vi "TrajectoryConfig_GetKinematicsMecanumDriveConstraint.vi"(11 "inTRAJECTORY_CONFIG":T1 {"End Velocity" format="%20.4f"; "StartVelocity" format="%20.4f"; "Max Acceleration" format="%20.4f"; "MaxVelocity" format="%20.4f"}) -> (1 "Constraint Exists":bool, 3 "Mecanum Drive Kinematics Constraint":T2={"Max Speed (M/S)"=0.0, "MECA_DRIVE_KINEMATICS"={"FrontLeft"={"X"=0.0, "Y"=0.0}, "FrontRight"={"X"=0.0, "Y"=0.0}, "RearLeft"={"X"=0.0, "Y"=0.0}, "RearRight"={"X"=0.0, "Y"=0.0}, "InverseKinematics"=[[0.0, 1.0, -1.0, 0.0], [0.0, 1.0, 1.0, 0.0], [0.0, 1.0, 1.0, 0.0], [0.0, 1.0, -1.0, 0.0]], "ForwardKinematics"=[[0.0, 1.0, -1.0, 0.0], [0.0, 1.0, 1.0, 0.0], [0.0, 1.0, 1.0, 0.0], [0.0, 1.0, -1.0, 0.0]], "PrevCoR"={"X"=0.0, "Y"=0.0}}} {"MECA_DRIVE_KINEMATICS"."PrevCoR"."Y" format="%14.3f"; "MECA_DRIVE_KINEMATICS"."PrevCoR"."X" format="%14.3f"; "MECA_DRIVE_KINEMATICS"."RearRight"."Y" format="%14.3f"; "MECA_DRIVE_KINEMATICS"."RearRight"."X" format="%14.3f"; "MECA_DRIVE_KINEMATICS"."RearLeft"."Y" format="%14.3f"; "MECA_DRIVE_KINEMATICS"."RearLeft"."X" format="%14.3f"; "MECA_DRIVE_KINEMATICS"."FrontRight"."Y" format="%14.3f"; "MECA_DRIVE_KINEMATICS"."FrontRight"."X" format="%14.3f"; "MECA_DRIVE_KINEMATICS"."FrontLeft"."Y" format="%14.3f"; "MECA_DRIVE_KINEMATICS"."FrontLeft"."X" format="%14.3f"; "Max Speed (M/S)" format="%20.4f"})   [LabVIEW 2019, in "Trajectory_Library.lvlib"]
doc: "Retrieves the Mecanum Kinematics constraint from the Trajectory Configuration.\n\nNote: If more than once instance of the Mecanum Kinematics constraint exists only the first one is returned. (Only one of these should be defined.)\n\nParameters:\n - InTrajectoryConfig -- The trajectory configuration data structure\n\nReturns:\n - Mecanum Kinematics Constraint -- The data cluster, which contains the constraint\n - Constraint Exists -- Returns TRUE if this constraint is defined in the trjaectory configuration."
uses:
  Trajectory_Library.lvlib
  TypeDef/TRAJ_CONSTRAINT_MECA_DRIVE_KINEMATICS.ctl
  TypeDef/MECA_DRIVE_KINEMATICS.ctl
  TypeDef/TRANSLATION2D.ctl
  <vilib>/Analysis/Matrix/Datatypes/RealMatrix.ctl
  TypeDef/TRAJ_CONFIG.ctl
  <vilib>/Utility/Data Type/NI_Data Type.lvlib
  <vilib>/Analysis/Matrix/NI_Matrix.lvlib
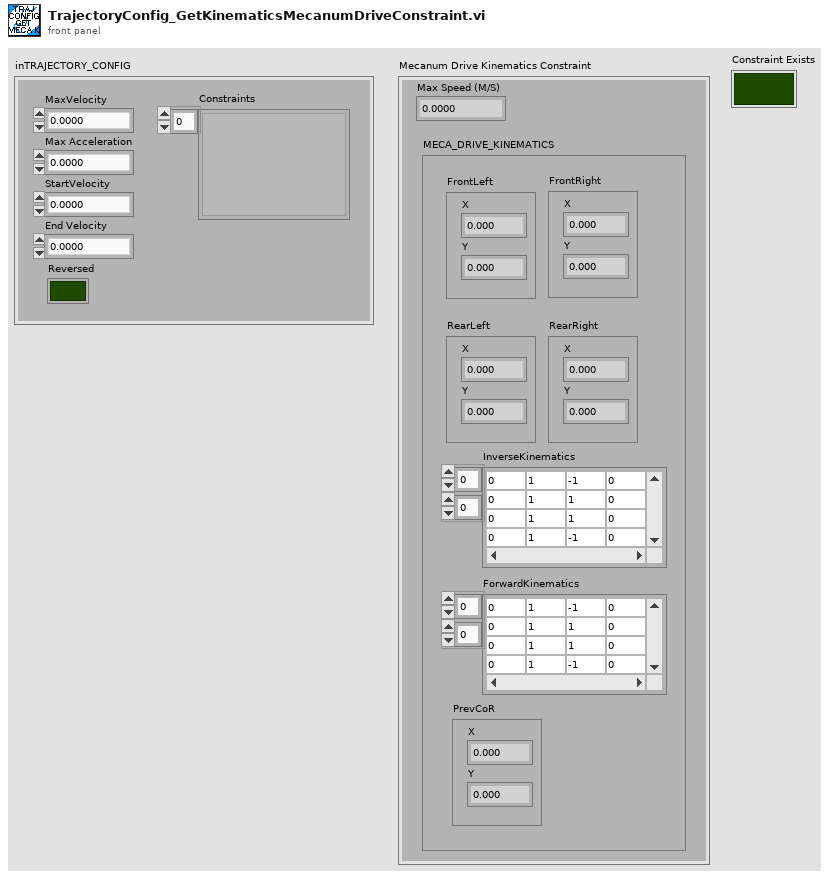
[diagram p1: front panel]
types:
  T1 = typedef "Trajectory_Library.lvlib/TRAJ_CONFIG.ctl" = cluster{"MaxVelocity":dbl, "Max Acceleration":dbl, "StartVelocity":dbl, "End Velocity":dbl, "Reversed":bool, "Constraints":variant[]}
  T2 = typedef "Trajectory_Library.lvlib/TRAJ_CONSTRAINT_MECA_DRIVE_KINEMATICS.ctl" = cluster{"Max Speed (M/S)":dbl, "MECA_DRIVE_KINEMATICS":T3}
  T3 = typedef "Trajectory_Library.lvlib/MECA_DRIVE_KINEMATICS.ctl" = cluster{"FrontLeft":T4, "FrontRight":T4, "RearLeft":T4, "RearRight":T4, "InverseKinematics":T5, "ForwardKinematics":T5, "PrevCoR":T4}
  T4 = typedef "Trajectory_Library.lvlib/TRANSLATION2D.ctl" = cluster{"X":dbl, "Y":dbl}
  T5 = typedef "NI_Matrix.lvlib/RealMatrix.ctl" = dbl[][]
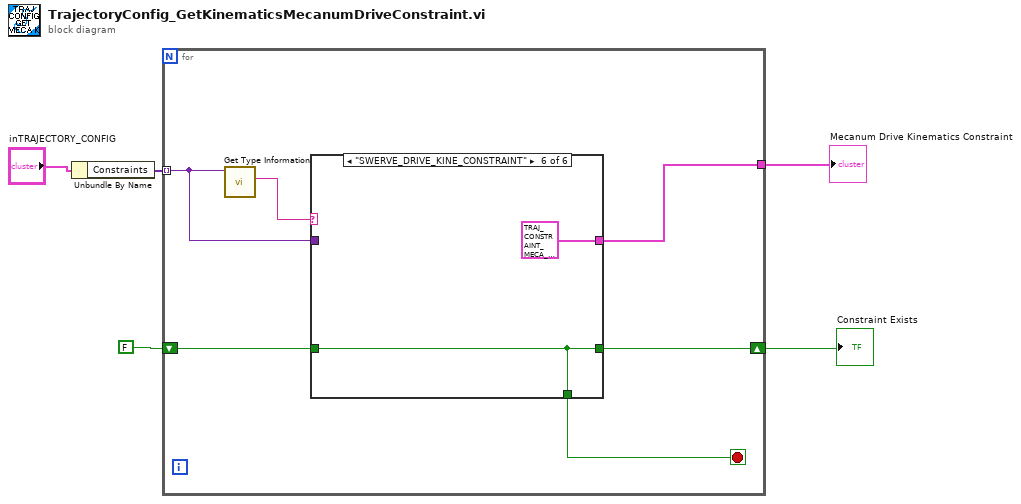
[diagram p0: block diagram]
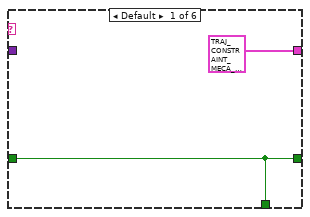
[diagram p2: hidden frame]
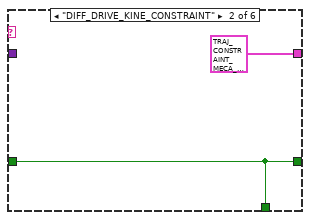
[diagram p3: hidden frame]
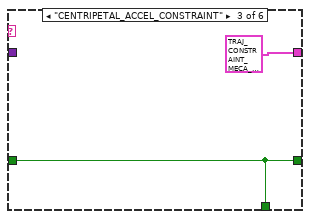
[diagram p4: hidden frame]
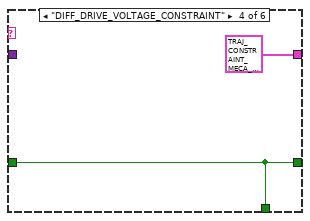
[diagram p5: hidden frame]
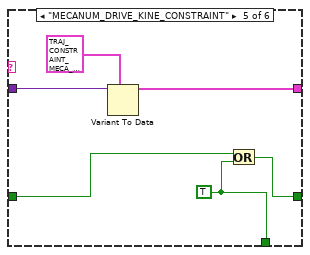
[diagram p6: hidden frame]
diagram:
  n1 = Unbundle By Name("inTRAJECTORY_CONFIG") -> ("Constraints"=w4:variant[])
  n2 = for {
    tunnel: w4 -> [w10] mode=indexing
    shift-right: [w8] -> w2
    shift-left: FALSE -> [w9]
    tunnel: [w6] -> w1
    stop <- w7 stop-if-true
    n3 = call <vilib>:"Get Type Information.vi"("variant"=w10) -> ("name"=w11:string)  [unwired: 6 in, 4 out]
    n4 = case shown="\"SWERVE_DRIVE_KINE_CONSTRAINT\"" w11 {
      tunnel: w10 -> [_ _ _ _ w24 _]
      tunnel: w9 -> [w13 w15 w17 w19 w21 w27]
      tunnel: [w13 w15 w17 w19 w23 w27] -> w8
      tunnel: [w13 w15 w17 w19 w22 w27] -> w7
      tunnel: [T2 {"Max Speed (M/S)"=0.0, "MECA_DRIVE_KINEMATICS"={"FrontLeft"={"X"=0.0, "Y"=0.0}, "FrontRight"={"X"=0.0, "Y"=0.0}, "RearLeft"={"X"=0.0, "Y"=0.0}, "RearRight"={"X"=0.0, "Y"=0.0}, "InverseKinematics"=[[0.0, 1.0, -1.0, 0.0], [0.0, 1.0, 1.0, 0.0], [0.0, 1.0, 1.0, 0.0], [0.0, 1.0, -1.0, 0.0]], "ForwardKinematics"=[[0.0, 1.0, -1.0, 0.0], [0.0, 1.0, 1.0, 0.0], [0.0, 1.0, 1.0, 0.0], [0.0, 1.0, -1.0, 0.0]], "PrevCoR"={"X"=0.0, "Y"=0.0}}} ("MECANUM_DRIVE_KINE_CONSTRAINT") T2 {"Max Speed (M/S)"=0.0, "MECA_DRIVE_KINEMATICS"={"FrontLeft"={"X"=0.0, "Y"=0.0}, "FrontRight"={"X"=0.0, "Y"=0.0}, "RearLeft"={"X"=0.0, "Y"=0.0}, "RearRight"={"X"=0.0, "Y"=0.0}, "InverseKinematics"=[[0.0, 1.0, -1.0, 0.0], [0.0, 1.0, 1.0, 0.0], [0.0, 1.0, 1.0, 0.0], [0.0, 1.0, -1.0, 0.0]], "ForwardKinematics"=[[0.0, 1.0, -1.0, 0.0], [0.0, 1.0, 1.0, 0.0], [0.0, 1.0, 1.0, 0.0], [0.0, 1.0, -1.0, 0.0]], "PrevCoR"={"X"=0.0, "Y"=0.0}}} ("MECANUM_DRIVE_KINE_CONSTRAINT") T2 {"Max Speed (M/S)"=0.0, "MECA_DRIVE_KINEMATICS"={"FrontLeft"={"X"=0.0, "Y"=0.0}, "FrontRight"={"X"=0.0, "Y"=0.0}, "RearLeft"={"X"=0.0, "Y"=0.0}, "RearRight"={"X"=0.0, "Y"=0.0}, "InverseKinematics"=[[0.0, 1.0, -1.0, 0.0], [0.0, 1.0, 1.0, 0.0], [0.0, 1.0, 1.0, 0.0], [0.0, 1.0, -1.0, 0.0]], "ForwardKinematics"=[[0.0, 1.0, -1.0, 0.0], [0.0, 1.0, 1.0, 0.0], [0.0, 1.0, 1.0, 0.0], [0.0, 1.0, -1.0, 0.0]], "PrevCoR"={"X"=0.0, "Y"=0.0}}} ("MECANUM_DRIVE_KINE_CONSTRAINT") T2 {"Max Speed (M/S)"=0.0, "MECA_DRIVE_KINEMATICS"={"FrontLeft"={"X"=0.0, "Y"=0.0}, "FrontRight"={"X"=0.0, "Y"=0.0}, "RearLeft"={"X"=0.0, "Y"=0.0}, "RearRight"={"X"=0.0, "Y"=0.0}, "InverseKinematics"=[[0.0, 1.0, -1.0, 0.0], [0.0, 1.0, 1.0, 0.0], [0.0, 1.0, 1.0, 0.0], [0.0, 1.0, -1.0, 0.0]], "ForwardKinematics"=[[0.0, 1.0, -1.0, 0.0], [0.0, 1.0, 1.0, 0.0], [0.0, 1.0, 1.0, 0.0], [0.0, 1.0, -1.0, 0.0]], "PrevCoR"={"X"=0.0, "Y"=0.0}}} ("MECANUM_DRIVE_KINE_CONSTRAINT") w20 T2 {"Max Speed (M/S)"=0.0, "MECA_DRIVE_KINEMATICS"={"FrontLeft"={"X"=0.0, "Y"=0.0}, "FrontRight"={"X"=0.0, "Y"=0.0}, "RearLeft"={"X"=0.0, "Y"=0.0}, "RearRight"={"X"=0.0, "Y"=0.0}, "InverseKinematics"=[[0.0, 1.0, -1.0, 0.0], [0.0, 1.0, 1.0, 0.0], [0.0, 1.0, 1.0, 0.0], [0.0, 1.0, -1.0, 0.0]], "ForwardKinematics"=[[0.0, 1.0, -1.0, 0.0], [0.0, 1.0, 1.0, 0.0], [0.0, 1.0, 1.0, 0.0], [0.0, 1.0, -1.0, 0.0]], "PrevCoR"={"X"=0.0, "Y"=0.0}}} ("MECANUM_DRIVE_KINE_CONSTRAINT")] -> w6
      frame Default {
      }
      frame "DIFF_DRIVE_KINE_CONSTRAINT" {
      }
      frame "CENTRIPETAL_ACCEL_CONSTRAINT" {
      }
      frame "DIFF_DRIVE_VOLTAGE_CONSTRAINT" {
      }
      frame "MECANUM_DRIVE_KINE_CONSTRAINT" {
        w22 = TRUE
        n5 = Variant To Data(type=T2 {"Max Speed (M/S)"=0.0, "MECA_DRIVE_KINEMATICS"={"FrontLeft"={"X"=0.0, "Y"=0.0}, "FrontRight"={"X"=0.0, "Y"=0.0}, "RearLeft"={"X"=0.0, "Y"=0.0}, "RearRight"={"X"=0.0, "Y"=0.0}, "InverseKinematics"=[[0.0, 1.0, -1.0, 0.0], [0.0, 1.0, 1.0, 0.0], [0.0, 1.0, 1.0, 0.0], [0.0, 1.0, -1.0, 0.0]], "ForwardKinematics"=[[0.0, 1.0, -1.0, 0.0], [0.0, 1.0, 1.0, 0.0], [0.0, 1.0, 1.0, 0.0], [0.0, 1.0, -1.0, 0.0]], "PrevCoR"={"X"=0.0, "Y"=0.0}}} ("MECANUM_DRIVE_KINE_CONSTRAINT"), Variant=w24) -> (data=w20:T2)  [unwired: 1 in, 1 out]
        n6 = Or(x=w21, y=w22) -> (x .or. y?=w23:bool)
      }
      frame "SWERVE_DRIVE_KINE_CONSTRAINT" {
      }
    }
  }
  "Mecanum Drive Kinematics Constraint" <- w1
  "Constraint Exists" <- w2
